vi "Configure Output.vi"(7 "Response  (0: Slow)":u16(ring) items=["Slow", "Fast"], 8 "error in (no error)":errorcluster, 9 "Output Mode  (0: DC)":u16(ring) items=["DC", "Pulse", "Sweep", "Pulse Sweep", "Pulse-RM"], 10 "Source Function  (0: Voltage)":u16(ring) items=["Voltage", "Current"], 11 "VISA resource name":refnum<visa-resource-name>) -> (0 "error out":errorcluster, 3 "VISA resource name out":refnum<visa-resource-name>)   [LabVIEW 2020, in "ADCMT 6240.lvlib"]
doc: "This VI configures source function and output mode."
uses:
  ADCMT 6240.lvlib
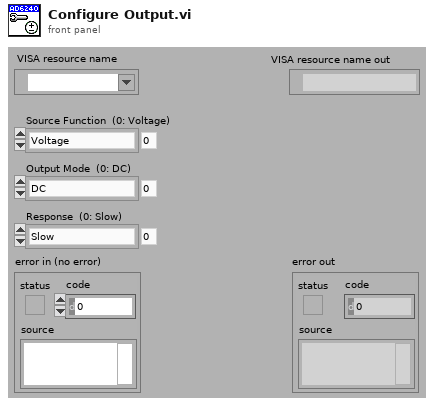
[diagram p1: front panel]
types:
  T1 = typedef "ADCMT 6240.lvlib/Extended User Data.ctl" = cluster{"Trigger Mode":u16, "Output Mode":u16, "Sample Count":i32, "Model":u16}
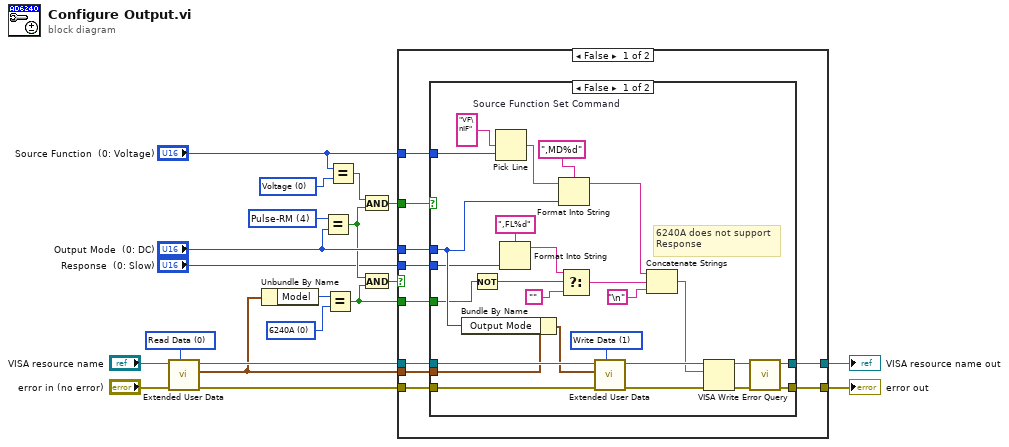
[diagram p0: block diagram]
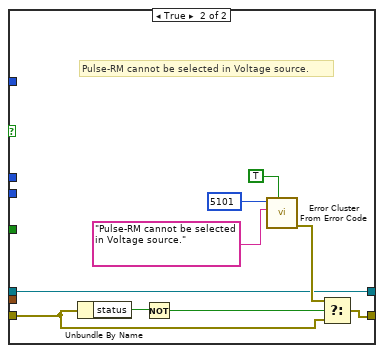
[diagram p2: hidden frame]
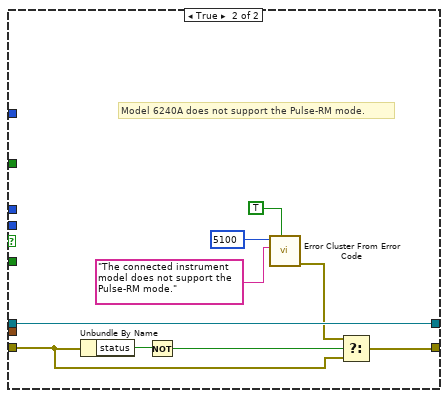
[diagram p3: hidden frame]
diagram:
  w10 = u16 0 items=["Voltage", "Current"] ("Source Function  (0: Voltage)")
  w5 = u16 4 items=["DC", "Pulse", "Sweep", "Pulse Sweep", "Pulse-RM"] ("Output Mode  (0: DC)")
  w11 = u16 0 items=["6240A", "6240B"] ("Model")
  w16 = u16 0 items=["Read Data", "Write Data", "Dispose of Data"] ("Action")
  n1 = call "Extended User Data.vi"("Action"=w16, "Error In (no error)"="error in (no error)", "VISA resource name in"="VISA resource name") -> ("Error Out"=w17:errorcluster, "User Data Out"=w13:T1, "VISA resource name out"=w18:refnum<visa-resource-name>)  [unwired: 6 in]
  n2 = Unbundle By Name(w13) -> ("Model"=w12:u16)
  n3 = Equal?(x=w5, y="Output Mode  (0: DC)") -> (x = y?=w3:bool)
  n4 = Equal?(x=w12, y=w11) -> (x = y?=w1:bool)
  n5 = Equal?(x="Source Function  (0: Voltage)", y=w10) -> (x = y?=w7:bool)
  n6 = And(x=w7, y=w3) -> (x .and. y?=w6:bool)
  n7 = And(x=w3, y=w1) -> (x .and. y?=w8:bool)
  n8 = case shown="False" w8 {
    tunnel: [w30 w68] -> w20
    tunnel: [w29 w72] -> w19
    tunnel: w18 -> [w28 w72]
    tunnel: w17 -> [w27 w69]
    tunnel: w13 -> [w26 _]
    tunnel: "Source Function  (0: Voltage)" -> [w25 _]
    tunnel: "Output Mode  (0: DC)" -> [w24 _]
    tunnel: w6 -> [w23 _]
    tunnel: "Response  (0: Slow)" -> [w22 _]
    tunnel: w1 -> [w21 _]
    frame False {
      n9 = case shown="False" w23 {
        tunnel: [w56 w60] -> w30
        tunnel: [w55 w59] -> w29
        tunnel: w28 -> [w51 w59]
        tunnel: w27 -> [w50 w61]
        tunnel: w26 -> [w44 _]
        tunnel: w25 -> [w43 _]
        tunnel: w24 -> [w40 _]
        tunnel: w22 -> [w37 _]
        tunnel: w21 -> [w35 _]
        frame False {
          w48 = u16 1 items=["Read Data", "Write Data", "Dispose of Data"] ("Action")
          w52 = "VF\nIF"  # Source Function Set Command
          # "6240A does not support Response"
          n10 = Bundle By Name(cluster=w44, "Output Mode"=w40) -> (w49:T1)
          n11 = Not(x=w35) -> (.not. x?=w33:bool)
          n12 = Pick Line(multi-line string=w52, line index=w43) -> (output string=w41:string)  [unwired: 1 in]
          n13 = Format Into String(format string=",FL%d", w37) -> (resulting string=w36:string)  [unwired: 2 in, 1 out]
          n14 = Format Into String(format string=",MD%d", initial string=w41, w40) -> (resulting string=w39:string)  [unwired: 1 in, 1 out]
          n15 = Select(t=w36, s=w33, f="") -> (s? t:f=w31:string)
          n16 = call "Extended User Data.vi"("Action"=w48, "Error In (no error)"=w50, "User Data In"=w49, "VISA resource name in"=w51) -> ("Error Out"=w46:errorcluster, "VISA resource name out"=w47:refnum<visa-resource-name>)  [unwired: 5 in, 1 out]
          n17 = Concatenate Strings(w39, w31, "\n") -> (w45:string)
          n18 = VISA Write(VISA resource name=w47, write buffer=w45, error in (no error)=w46) -> (VISA resource name out=w54:refnum<visa-resource-name>, error out=w53:errorcluster)  [unwired: 1 out]
          n19 = call "Error Query.vi"("error in (no error)"=w53, "VISA resource name"=w54) -> ("error out"=w56:errorcluster, "VISA resource name out"=w55:refnum<visa-resource-name>)  [unwired: 6 in, 2 out]
        }
        frame True {
          # "Pulse-RM cannot be selected in Voltage source."
          n20 = Unbundle By Name(w61) -> ("status"=w58:bool)
          n21 = Not(x=w58) -> (.not. x?=w63:bool)
          n22 = call <vilib>:"Error Cluster From Error Code.vi"("show call chain? (False)"=TRUE, "error message (\"\")"="Pulse-RM cannot be selected in Voltage source." ("Source (VI Name)"), "error code (0)"=5101 ("Code")) -> ("error out"=w62:errorcluster)  [unwired: 6 in]
          n23 = Select(t=w62, s=w63, f=w61) -> (s? t:f=w60:errorcluster)
        }
      }
    }
    frame True {
      # "Model 6240A does not support the Pulse-RM mode."
      n24 = Unbundle By Name(w69) -> ("status"=w71:bool)
      n25 = Not(x=w71) -> (.not. x?=w70:bool)
      n26 = call <vilib>:"Error Cluster From Error Code.vi"("show call chain? (False)"=TRUE, "error message (\"\")"="The connected instrument model does not support the Pulse-RM mode." ("Source (VI Name)"), "error code (0)"=5100 ("Code")) -> ("error out"=w67:errorcluster)  [unwired: 6 in]
      n27 = Select(t=w67, s=w70, f=w69) -> (s? t:f=w68:errorcluster)
    }
  }
  "error out" <- w20
  "VISA resource name out" <- w19
